vi "ComputeDesiredState.vi"(11 "Robot Action Array":T1[](array[typedef])) -> ()   [LabVIEW 2018]
uses:
  Controls/Robot Actions.ctl
  Controls/Robot State.ctl
  Controls/Robot Pivot Motion Commands.ctl
  Controls/Pivot Motor Commands.ctl
  Controls/Robot Drive Mode.ctl
  Controls/Climb Motor Commands.ctl
  Controls/Arm Motor Commands.ctl
  Controls/Ball Motor Commands.ctl
  Controls/Dics Eject Command.ctl
  Controls/Lift Motor Commands.ctl
  Controls/Grip Motor Commands.ctl
  Controls/Enable Actions.ctl
  Global Variables/Trajectory Enabled.vi
  Global Variables/Robot State.vi
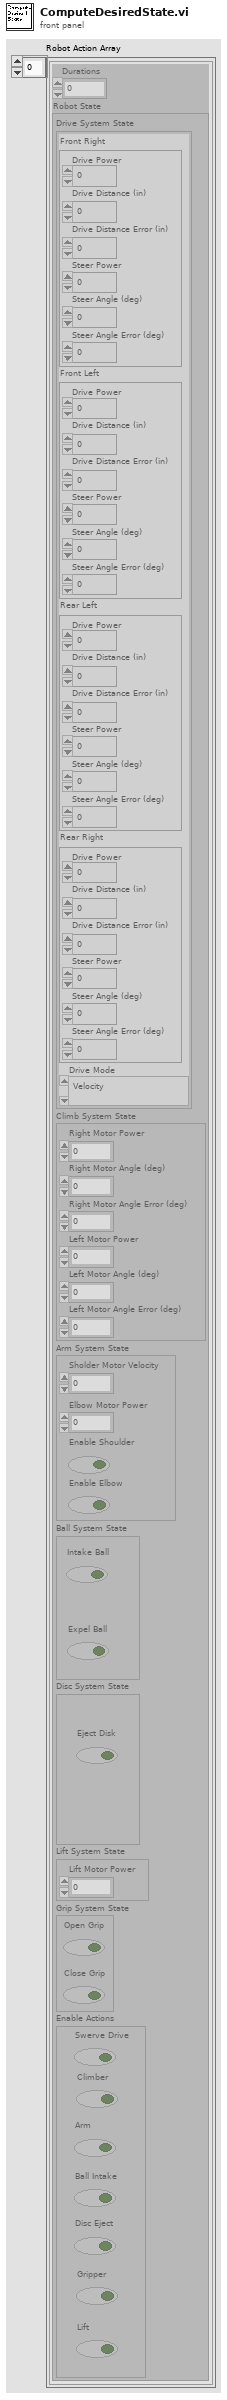
[diagram p1: front panel]
types:
  T1 = typedef "Robot Actions.ctl" = cluster{"Durations":dbl, "Robot State":T2}
  T2 = typedef "Robot State.ctl" = cluster{"Drive System State":T3, "Climb System State":T6, "Arm System State":T7, "Ball System State":T8, "Disc System State":T9, "Lift System State":T10, "Grip System State":T11, "Enable Actions":T12}
  T3 = typedef "Robot Pivot Motion Commands.ctl" = cluster{"Front Right":T4, "Front Left":T4, "Rear Left":T4, "Rear Right":T4, "Drive Mode":T5}
  T4 = typedef "Pivot Motor Commands.ctl" = cluster{"Drive Power":dbl, "Drive Distance (in)":dbl, "Drive Distance Error (in)":dbl, "Steer Power":dbl, "Steer Angle (deg)":dbl, "Steer Angle Error (deg)":dbl}
  T5 = typedef "Robot Drive Mode.ctl" = enum16{"Velocity", "Distance"}
  T6 = typedef "Climb Motor Commands.ctl" = cluster{"Right Motor Power":dbl, "Right Motor Angle (deg)":dbl, "Right Motor Angle Error (deg)":dbl, "Left Motor Power":dbl, "Left Motor Angle (deg)":dbl, "Left Motor Angle Error (deg)":dbl}
  T7 = typedef "Arm Motor Commands.ctl" = cluster{"Enable Shoulder":bool, "Enable Elbow":bool, "Elbow Motor Power":dbl, "Sholder Motor Velocity":dbl}
  T8 = typedef "Ball Motor Commands.ctl" = cluster{"Intake Ball":bool, "Expel Ball":bool}
  T9 = typedef "Dics Eject Command.ctl" = cluster{"Eject Disk":bool}
  T10 = typedef "Lift Motor Commands.ctl" = cluster{"Lift Motor Power":dbl}
  T11 = typedef "Grip Motor Commands.ctl" = cluster{"Open Grip":bool, "Close Grip":bool}
  T12 = typedef "Enable Actions.ctl" = cluster{"Swerve Drive":bool, "Climber":bool, "Arm":bool, "Ball Intake":bool, "Disc Eject":bool, "Gripper":bool, "Lift":bool}
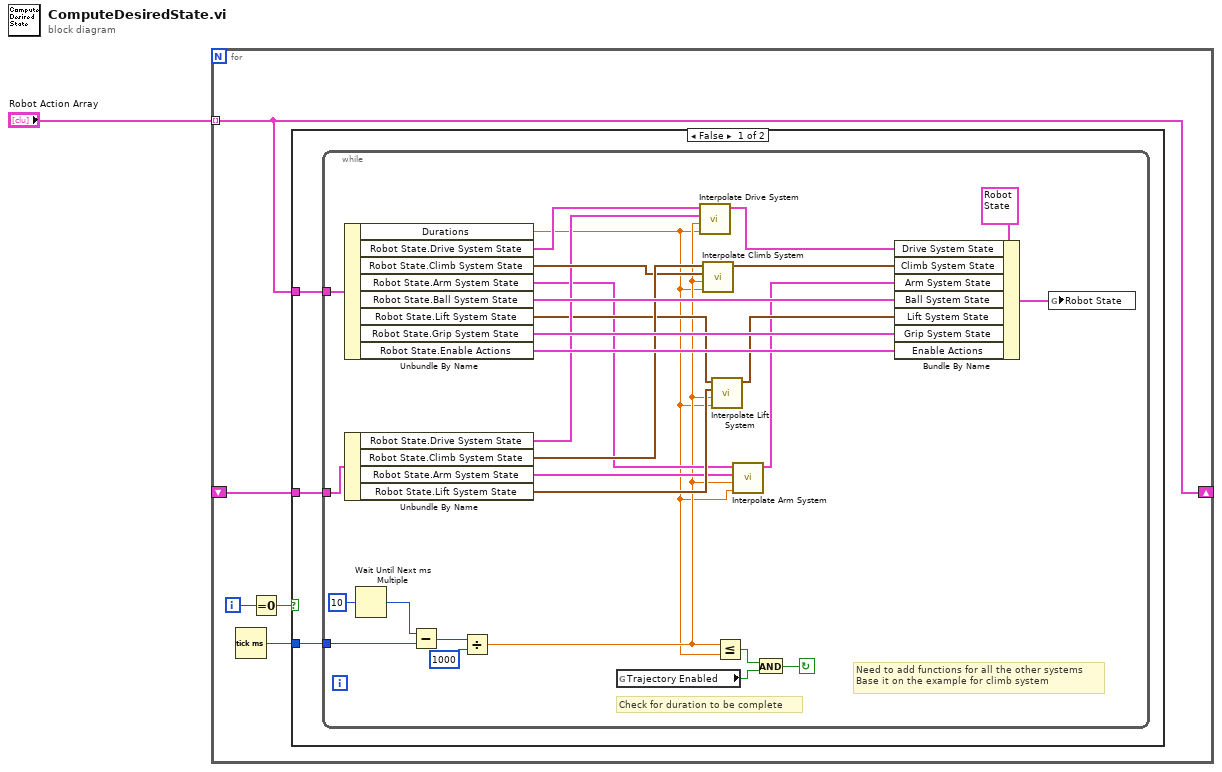
[diagram p0: block diagram]
diagram:
  n1 = for {
    tunnel: "Robot Action Array" -> [w3] mode=indexing
    shift-right: [w3] -> _
    shift-left: _ -> [w4]
    i -> [w6]
    n2 = Tick Count (ms)() -> (millisecond timer value=w2:u32)
    n3 = Equal To 0?(x=w6) -> (x = 0?=w5:bool)
    n4 = case shown="False" w5 {
      tunnel: w4 -> [w8 _]
      tunnel: w3 -> [w9 _]
      tunnel: w2 -> [w7 _]
      frame False {
        n5 = while {
          tunnel: w9 -> [w37]
          tunnel: w8 -> [w38]
          tunnel: w7 -> [w31]
          stop <- w26 continue-if-true
          # "Need to add functions for all the other systems\nBase it on the example for climb system"
          # "Check for duration to be complete"
          n6 = Unbundle By Name(w37) -> ("Durations"=w10:dbl, "Robot State.Drive System State"=w19:T3, "Robot State.Climb System State"=w21:T6, "Robot State.Arm System State"=w14:T7, "Robot State.Ball System State"=w24:T8, "Robot State.Lift System State"=w17:T10, "Robot State.Grip System State"=w23:T11, "Robot State.Enable Actions"=w34:T12)
          n7 = Unbundle By Name(w38) -> ("Robot State.Drive System State"=w20:T3, "Robot State.Climb System State"=w22:T6, "Robot State.Arm System State"=w13:T7, "Robot State.Lift System State"=w15:T10)
          n8 = Wait Until Next ms Multiple(millisecond multiple=u32 10) -> (millisecond timer value=w32:u32)
          n9 = Subtract(x=w32, y=w31) -> (x-y=w30:u32)
          n10 = Divide(x=w30, y=u32 1000) -> (x/y=w11:dbl)
          n11 = global read "Trajectory Enabled.vi" "Trajectory Enabled"() -> (w27:bool)
          n12 = call "Interpolate Drive System.vi"("Duration"=w10, "Current Time"=w11, "Start Robot Commands"=w20, "End Robot Commands"=w19) -> ("Current Robot Commands"=w18:T3)  [unwired: 7 in]
          n13 = call "Interpolate Climb System.vi"("Duration"=w10, "Current Time"=w11, "End Climb Motor Commands"=w21, "Start Climb Motor Commands"=w22) -> ("Current Climb Motor Commands"=w33:T6)  [unwired: 7 in]
          n14 = call "Interpolate Lift System.vi"("Duration"=w10, "Current Time"=w11, "Start Lift Motor Commands"=w15, "End Lift Motor Commands"=w17) -> ("Current Lift Motor Commands"=w16:T10)  [unwired: 7 in]
          n15 = Less Or Equal?(x=w11, y=w10) -> (x <= y?=w28:bool)
          n16 = call "Interpolate Arm System.vi"("Duration"=w10, "Current Time"=w11, "Start Arm Motor Commands"=w13, "End Arm Motor Commands"=w14) -> ("Current Arm Motor Commands"=w12:T7)  [unwired: 7 in]
          n17 = And(x=w28, y=w27) -> (x .and. y?=w26:bool)
          n18 = Bundle By Name(cluster=T2 {"Drive System State"={"Front Right"={"Drive Power"=0.0, "Drive Distance (in)"=0.0, "Drive Distance Error (in)"=0.0, "Steer Power"=0.0, "Steer Angle (deg)"=0.0, "Steer Angle Error (deg)"=0.0}, "Front Left"={"Drive Power"=0.0, "Drive Distance (in)"=0.0, "Drive Distance Error (in)"=0.0, "Steer Power"=0.0, "Steer Angle (deg)"=0.0, "Steer Angle Error (deg)"=0.0}, "Rear Left"={"Drive Power"=0.0, "Drive Distance (in)"=0.0, "Drive Distance Error (in)"=0.0, "Steer Power"=0.0, "Steer Angle (deg)"=0.0, "Steer Angle Error (deg)"=0.0}, "Rear Right"={"Drive Power"=0.0, "Drive Distance (in)"=0.0, "Drive Distance Error (in)"=0.0, "Steer Power"=0.0, "Steer Angle (deg)"=0.0, "Steer Angle Error (deg)"=0.0}, "Drive Mode"=enum."Velocity"}, "Climb System State"={"Right Motor Power"=0.0, "Right Motor Angle (deg)"=0.0, "Right Motor Angle Error (deg)"=0.0, "Left Motor Power"=0.0, "Left Motor Angle (deg)"=0.0, "Left Motor Angle Error (deg)"=0.0}, "Arm System State"={"Enable Shoulder"=FALSE, "Enable Elbow"=FALSE, "Elbow Motor Power"=0.0, "Sholder Motor Velocity"=0.0}, "Ball System State"={"Intake Ball"=FALSE, "Expel Ball"=FALSE}, "Disc System State"={"Eject Disk"=FALSE}, "Lift System State"={"Lift Motor Power"=0.0}, "Grip System State"={"Open Grip"=FALSE, "Close Grip"=FALSE}, "Enable Actions"={"Swerve Drive"=FALSE, "Climber"=FALSE, "Arm"=FALSE, "Ball Intake"=FALSE, "Disc Eject"=FALSE, "Gripper"=FALSE, "Lift"=FALSE}} ("Robot State"), "Drive System State"=w18, "Climb System State"=w33, "Arm System State"=w12, "Ball System State"=w24, "Lift System State"=w16, "Grip System State"=w23, "Enable Actions"=w34) -> (w35:T2)
          n19 = global write "Robot State.vi" "Robot State"(w35) -> ()
        }
      }
      frame True {
        # "Ignore the first time through the loop because it is the starting point for the trajectory."
      }
    }
  }
